vi "Toolkit Binaries Post-Install Custom Action.vi"(10 "Variant":variant) -> (0 "error out":errorcluster)   [LabVIEW 2020]
uses:
  binary_installation_tools/binary_installation_tools.lvlib
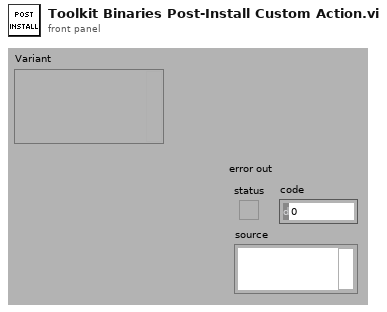
[diagram p1: front panel]
types:
  T1 = typedef "binary_installation_tools.lvlib/Binary Dependency Platform.ctl" = enum16{"Windows Desktop x86", "Windows Desktop x64", "Linux Desktop x64", "Linux Desktop aarch64", "NI Linux RT x64", "NI Linux RT armv7a"}
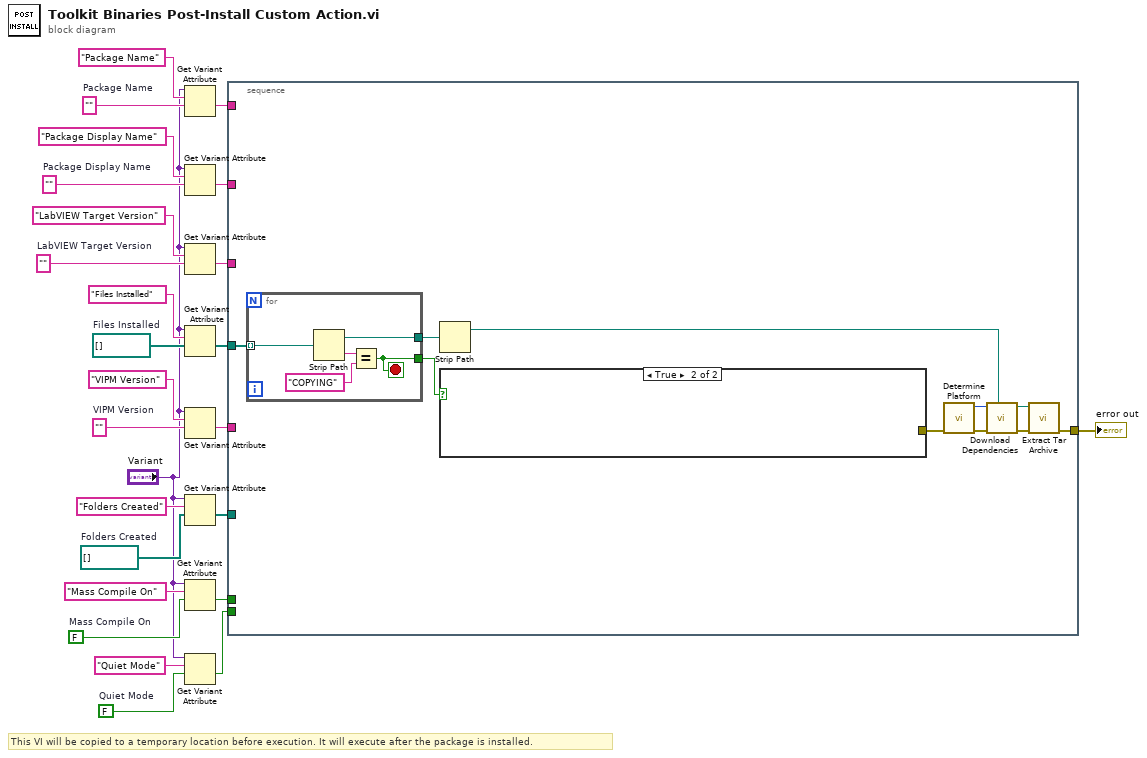
[diagram p0: block diagram]
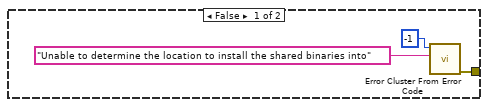
[diagram p2: hidden frame]
diagram:
  w3 = path[] []  # Folders Created
  w4 = path[] []  # Files Installed
  w9 = FALSE  # Mass Compile On
  w10 = ""  # Package Display Name
  w17 = FALSE  # Quiet Mode
  w20 = ""  # VIPM Version
  w22 = ""  # LabVIEW Target Version
  w24 = ""  # Package Name
  # "This VI will be copied to a temporary location before execution. It will execute after the package is installed."
  n1 = Get Variant Attribute(Variant="Variant", name="Package Name", default value (empty Variant)=w24) -> (value=w15:string)  [unwired: 1 in, 3 out]
  n2 = Get Variant Attribute(Variant="Variant", name="Package Display Name", default value (empty Variant)=w10) -> (value=w16:string)  [unwired: 1 in, 3 out]
  n3 = Get Variant Attribute(Variant="Variant", name="LabVIEW Target Version", default value (empty Variant)=w22) -> (value=w14:string)  [unwired: 1 in, 3 out]
  n4 = Get Variant Attribute(Variant="Variant", name="Files Installed", default value (empty Variant)=w4) -> (value=w6:path[])  [unwired: 1 in, 3 out]
  n5 = Get Variant Attribute(Variant="Variant", name="VIPM Version", default value (empty Variant)=w20) -> (value=w13:string)  [unwired: 1 in, 3 out]
  n6 = Get Variant Attribute(Variant="Variant", name="Folders Created", default value (empty Variant)=w3) -> (value=w7:path[])  [unwired: 1 in, 3 out]
  n7 = Get Variant Attribute(Variant="Variant", name="Mass Compile On", default value (empty Variant)=w9) -> (value=w11:bool)  [unwired: 1 in, 3 out]
  n8 = Get Variant Attribute(Variant="Variant", name="Quiet Mode", default value (empty Variant)=w17) -> (value=w12:bool)  [unwired: 1 in, 3 out]
  n9 = stacked-sequence {
    tunnel: w16 -> [_]
    tunnel: w15 -> [_]
    tunnel: w14 -> [_]
    tunnel: w13 -> [_]
    tunnel: w12 -> [_]
    tunnel: w11 -> [_]
    tunnel: w6 -> [w31]
    tunnel: w7 -> [_]
    tunnel: [w32] -> w1
    frame #0 {
      n10 = for {
        tunnel: w31 -> [w44] mode=indexing
        tunnel: [w41] -> w30
        tunnel: [w40] -> w28
        stop <- w40 stop-if-true
        n11 = Strip Path(path=w44) -> (stripped path=w41:path, name=w43:string)
        n12 = Equal?(x=w43, y="COPYING") -> (x = y?=w40:bool)
      }
      n13 = Strip Path(path=w30) -> (stripped path=w29:path)  [unwired: 1 out]
      n14 = case shown="True" w28 {
        tunnel: [w39 _] -> w27
        frame False {
          n15 = call <vilib>:"Error Cluster From Error Code.vi"("error message (\"\")"="Unable to determine the location to install the shared binaries into" ("error message (\"\")"), "error code (0)"=-1) -> ("error out"=w39:errorcluster)  [unwired: 7 in]
        }
        frame True {
        }
      }
      n16 = call "Determine Platform.vi"("error in (no error)"=w27) -> ("error out"=w35:errorcluster, "Platform"=w36:T1)  [unwired: 9 in]
      n17 = call "Download Dependencies.vi"("Target Directory"=w29, "error in (no error)"=w35, "Platform"=w36) -> ("error out"=w33:errorcluster, "Downloaded File"=w34:path)  [unwired: 7 in]
      n18 = call "Extract Tar Archive.vi"("error in (no error)"=w33, "File"=w34) -> ("error out"=w32:errorcluster)  [unwired: 9 in]
    }
  }
  "error out" <- w1
